vi "Set-Exposure-mode.vi"(8 "error in (no error)":errorcluster, 10 "Acquis. params. ref. in":refnum<data-value>, 11 "PF_MV1-D1312-240 in":refnum<class "PF_MV1-D1312-240.lvclass">) -> (0 "error out":errorcluster, 2 "Acquis. params. ref.":refnum<data-value>, 3 "PF_MV1-D1312-240 out":refnum<class "PF_MV1-D1312-240.lvclass">)   [LabVIEW 2013, in "CameraVision.lvlib" / "PF_MV1-D1312-240.lvclass"]
uses:
  PF_MV1-D1312-240.lvclass
  Main/Acquisition/CV-Acquisition.lvclass
  Camera.lvclass/Camera.ctl
  Main/Acquisition/CV-Acquisition.lvclass/CV-Acquisition.ctl
  Main/Acquisition/Read Exposure mode.vi
  Main/Acquisition/Read Value 1.vi
  Main/Acquisition/Read Value 2.vi
  Main/Acquisition/Read Time 1.vi
  Main/Acquisition/Read Time 2.vi
  <userlib>/Photonfocus Toolkit/_Public/SubVIs/pf_Set_Camera_Property_Mode.vi
  <userlib>/Photonfocus Toolkit/_Public/SubVIs/pf_Set_Camera_Property_Int.vi
  <userlib>/Photonfocus Toolkit/Photonfocus_Toolkit.lvlib
  Camera.lvclass
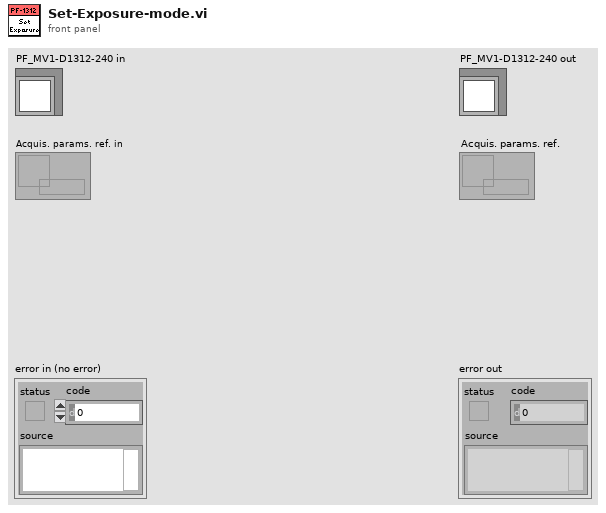
[diagram p1: front panel]
types:
  T1 = typedef "CameraVision.lvlib/Acquisition.lvclass/Exposure-modes.ctl" = enum16{"Linear", "LinLog"}
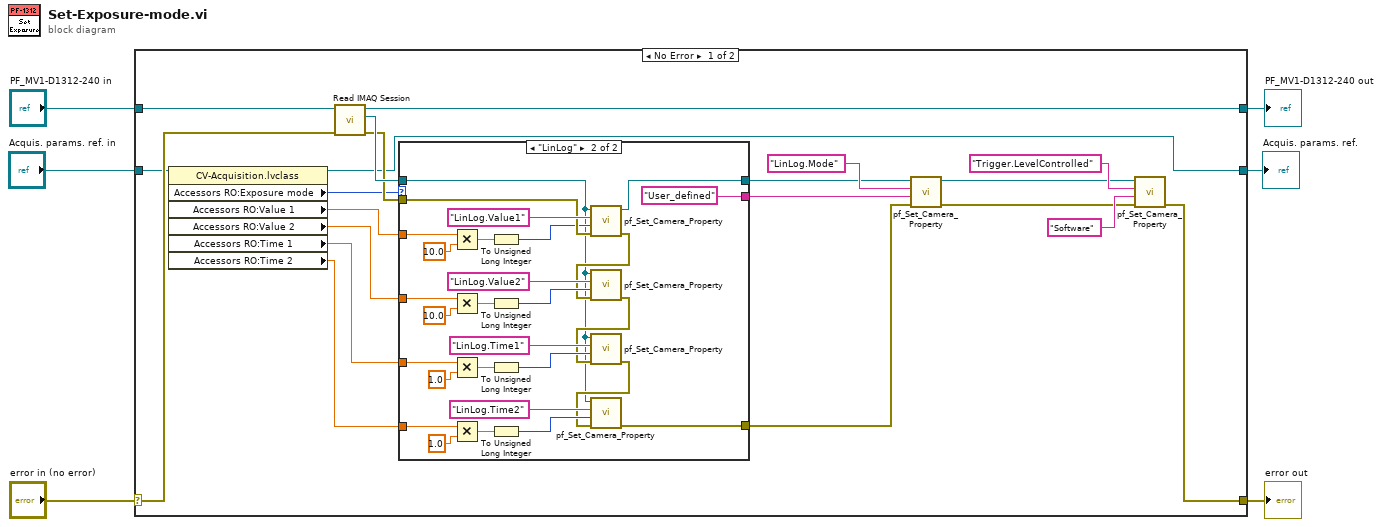
[diagram p0: block diagram]
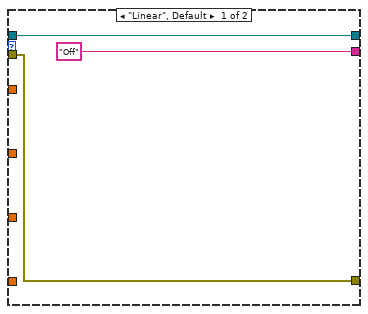
[diagram p2: hidden frame]
diagram:
  n1 = case shown="No Error" "error in (no error)" {
    selector: "error in (no error)" -> [w25 w61]
    tunnel: [w14 w61] -> w5
    tunnel: [w26 w60] -> w3
    tunnel: "PF_MV1-D1312-240 in" -> [w27 w60]
    tunnel: "Acquis. params. ref. in" -> [w13 w59]
    tunnel: [w7 w59] -> w1
    frame No Error {
      n2 = property class="CV-Acquisition.lvclass"(reference=w13) -> (reference out=w7:refnum<data-value>, "Accessors RO:Exposure mode"=w12:T1, "Accessors RO:Value 1"=w11:dbl, "Accessors RO:Value 2"=w10:dbl, "Accessors RO:Time 1"=w9:dbl, "Accessors RO:Time 2"=w8:dbl)  [unwired: 1 in, 1 out]
      n3 = call "Read IMAQ Session.vi"("error in (no error)"=w25, "Camera in"=w27) -> ("error out"=w17:errorcluster, "IMAQ Session"=w19:refnum<k11>, "Camera out"=w26:refnum<class "PF_MV1-D1312-240.lvclass">)  [unwired: 7 in]
      n4 = case shown="\"LinLog\"" w12 {
        tunnel: ["Off" "User_defined"] -> w23
        tunnel: w19 -> [w29 w32]
        tunnel: w8 -> [_ w34]
        tunnel: w9 -> [_ w40]
        tunnel: w10 -> [_ w47]
        tunnel: w11 -> [_ w55]
        tunnel: w17 -> [w28 w56]
        tunnel: [w29 w33] -> w18
        tunnel: [w28 w31] -> w16
        frame "Linear", Default {
        }
        frame "LinLog" {
          n5 = Multiply(x=w55, y=10.0) -> (x*y=w53:dbl)
          n6 = Multiply(x=w47, y=10.0) -> (x*y=w49:dbl)
          n7 = Multiply(x=w40, y=1.0) -> (x*y=w43:dbl)
          n8 = Multiply(x=w34, y=1.0) -> (x*y=w37:dbl)
          n9 = To Unsigned Long Integer(number=w53) -> (unsigned 32bit integer=w52:u32)
          n10 = To Unsigned Long Integer(number=w49) -> (unsigned 32bit integer=w48:u32)
          n11 = To Unsigned Long Integer(number=w43) -> (unsigned 32bit integer=w42:u32)
          n12 = To Unsigned Long Integer(number=w37) -> (unsigned 32bit integer=w36:u32)
          n13 = call-poly <userlib>:"pf_Set_Camera_Property.vi"("error in (no error)"=w56, "Property Value"=w52, "Property Name"="LinLog.Value1", "IMAQ Session in"=w32) -> ("error out"=w46:errorcluster, "IMAQ Session out"=w33:refnum<k11>)  [unwired: 5 in, 1 out]
          n14 = call-poly <userlib>:"pf_Set_Camera_Property.vi"("error in (no error)"=w46, "Property Value"=w48, "Property Name"="LinLog.Value2", "IMAQ Session in"=w32) -> ("error out"=w41:errorcluster)  [unwired: 5 in, 2 out]
          n15 = call-poly <userlib>:"pf_Set_Camera_Property.vi"("error in (no error)"=w41, "Property Value"=w42, "Property Name"="LinLog.Time1", "IMAQ Session in"=w32) -> ("error out"=w35:errorcluster)  [unwired: 5 in, 2 out]
          n16 = call-poly <userlib>:"pf_Set_Camera_Property.vi"("error in (no error)"=w35, "Property Value"=w36, "Property Name"="LinLog.Time2", "IMAQ Session in"=w32) -> ("error out"=w31:errorcluster)  [unwired: 5 in, 2 out]
        }
      }
      n17 = call-poly <userlib>:"pf_Set_Camera_Property.vi"("error in (no error)"=w16, "Property Value"=w23, "Property Name"="LinLog.Mode", "IMAQ Session in"=w18) -> ("error out"=w15:errorcluster, "IMAQ Session out"=w20:refnum<k11>)  [unwired: 5 in, 1 out]
      n18 = call-poly <userlib>:"pf_Set_Camera_Property.vi"("error in (no error)"=w15, "Property Value"="Software", "Property Name"="Trigger.LevelControlled", "IMAQ Session in"=w20) -> ("error out"=w14:errorcluster)  [unwired: 5 in, 2 out]
    }
    frame Error {
    }
  }
  "error out" <- w5
  "PF_MV1-D1312-240 out" <- w3
  "Acquis. params. ref." <- w1
